vi "Find Device Name.vi"(11 "Device Type":string="PCIe-6343") -> (3 "Device Name":string)   [LabVIEW 2015]
uses:
  <resource>/objmgr/daqmx.rc
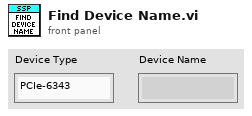
[diagram p1: front panel]
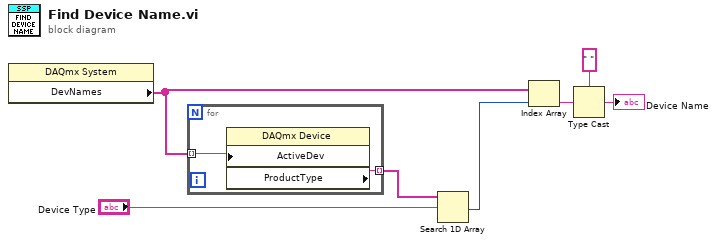
[diagram p0: block diagram]
diagram:
  n1 = property class="DAQmx System"() -> ("DevNames"=w5:tag[])  [unwired: 2 in, 2 out]
  n2 = for {
    tunnel: w5 -> [w9] mode=indexing
    tunnel: [w8] -> w7 mode=indexing
    n3 = property class="DAQmx Device"("ActiveDev"=w9) -> ("ProductType"=w8:string)  [unwired: 2 in, 2 out]
  }
  n4 = Search 1D Array(1D array=w7, element="Device Type") -> (index of element=w4:i32)  [unwired: 1 in]
  n5 = Index Array(array=w5, index=w4) -> (element=w3:tag)
  n6 = Type Cast(type=" ", x=w3) -> (*(type *) &x=→"Device Name":string)
